vi "experiment control.vi"() -> ()   [LabVIEW 2012] (continued)
  in  "Functions":cluster{"Name":string, "Body":string}[](array[cluster])=[{"Name"="Warmup Ablation Laser", "Body"="Debug: Console >> Start Warmup\nDIO64: Prepare >> Experiment\nFrames >> 50,1\nDIO64: Run\nDebug: Console >> End Warmup"}, {"Name"="Read Wavelengths", "Body"="Wavemeter: Read\nLaser: Read Wavelength >> Lisa"}, {"Name"="scan", "Body"="Begin Scan\n\nScan: Reference >> Disable,All\n\n#Scan: Reference >> Enable,0\n#Scan: Reference >> Enable,1\n#Scan: Reference >> Enable,2\n#Scan: Reference >> Enable,3\n#Scan: Reference >> Enable,4\n#Scan: Reference >> Enable,5\n#Scan: Reference >> Enable,6\n#Scan: Reference >> Enable,7\nScan: Reference >> Enable,8\nScan: Reference >> Enable,9\nScan: Reference >> Enable,10\n\n#Scan: Reset >>0\n#Scan: Reset >>1\n#Scan: Reset >>2\nScan: Reset >>3\n\nFrames  >> 40,40\nScope: Settings >> TDS5034B\nScope: Trigger Settings >> TDS5034B\n\nWhile Loop >> Scan\nTrap DDS: Upload\n\nDAC: Upload2 >> 0,Fast\nFor Loop >> 3\n\nMacro: Clear Wavelengths\nMacro: Read Wavelengths\nQuadDVM: Read\n\nScope: Start >> TDS5034B\nDIO64: Run >> Chop,0\nScope: Read >> TDS5034B\nScope: Stop >> TDS5034B\nScope: Display Traces >> TDS5034B\n\nubinary2 >> Save Scan\n\nEnd Loop\n\n#Scan: Step >>0\n#Scan: Step >>1\n#Scan: Step >>2\nScan: Step >>3\nEnd Loop"}, {"Name"="Scan Experiment Trap Time", "Body"="Frames >> 3,3\nScope: Settings >> TDS5034B\nScope: Trigger Settings >> TDS5034B\n\nBegin Scan\nScan: Reference >> Disable,All\nScan: Reference >> Enable,8\nScan: Reset >> 0\n\nWhile Loop >> Scan\nMacro: Clear Wavelengths\nMacro: Read Wavelengths\n\nScope: Start >> TDS5034B\n\nMV500: Trigger >> True\nDAC: Upload2 >> 1,IMG\nDIO64: Prepare >> 6\nDIO64: Run\nDAC: Upload2 >> 1,Fast\nDIO64: Prepare >> 5\nDIO64: Run\n\nScope: Read >> TDS5034B\nScope: Stop >> TDS5034B\n\nScope: Display Traces >> TDS5034B\nMacro: Read Wavelengths\nuBinary2 >> Save Scan\nScan: Step >> 0\nEnd Loop"}, {"Name"="Scan LIF", "Body"="Frames >> 100, 200\nScope: Settings >> TDS5034B\nScope: Trigger Settings >> TDS5034B\n\nBegin Scan\n\nFor Loop >> 200\nMacro: Clear Wavelengths\nMacro: Read Wavelengths\nScope: Start >> TDS5034B\n#DIO64: Prepare >> Experiment 2-color Photodissoc\nDIO64: Run >> Chop\nScope: Read >> TDS5034B\nScope: Stop >> TDS5034B\nScope: Display Traces >> TDS5034B\nMacro: Read Wavelengths\nuBinary >> Save Scan\nEnd Loop"}, {"Name"="Check ion number", "Body"="Frames >> 30,30\nScope: Settings >> TDS5034B\nScope: Trigger Settings >> TDS5034B\n\nBegin Scan\n\nFor Loop >> 10\nMacro: Clear Wavelengths\nMacro: Read Wavelengths\nCounter: Read\n\nScope: Start >> TDS5034B\nDIO64: Run >> Chop,1\nScope: Read >> TDS5034B\nScope: Stop >> TDS5034B\n\nScope: Display Traces >> TDS5034B\nubinary2 >> Save Scan\nEnd Loop\n"}, {"Name"="Scan Cora", "Body"="Go Today\nMove Down >> scan_cora\n\nFrames >> 15,15\nScope: Settings >> TDS5034B\nScope: Trigger Settings >> TDS5034B\n\nBegin Scan\nLaser: Start Scan >> Cora\nLaser: Step Wavelength >> Cora\nMacro: Read Wavelengths\nWhile Loop >> Cora\nFor Loop >> 3\n\nMacro: Clear Wavelengths\nMacro: Read Wavelengths\nScope: Start >> TDS5034B\nDIO64: Run >> Chop,0\nScope: Read >> TDS5034B\nScope: Stop >> TDS5034B\nScope: Display Traces >> TDS5034B\nMacro: Read Wavelengths\nuBinary: Save\n\nEnd Loop\n\nLaser: Step Wavelength >> Cora\n\nEnd Loop"}, {"Name"="Scan Bertha", "Body"="Frames >> 30,30\nScope: Settings >> TDS5034B\nScope: Trigger Settings >> TDS5034B\n\nBegin Scan\nLaser: Start Scan >> Bertha\nLaser: Step Wavelength >> Bertha\nMacro: Read Wavelengths\nWhile Loop >> Bertha\nFor Loop >> 3\n\nMacro: Clear Wavelengths\nMacro: Read Wavelengths\nScope: Start >> TDS5034B\nDIO64: Run >> Chop,0\nScope: Read >> TDS5034B\nScope: Stop >> TDS5034B\nScope: Display Traces >> TDS5034B\nMacro: Read Wavelengths\nuBinary2 >> Save Scan\n\nEnd Loop\n\nLaser: Step Wavelength >> Bertha\n\nEnd Loop"}, {"Name"="Scan Laser", "Body"="Frames >> 120,120\nScope: Settings >> TDS5034B\nScope: Trigger Settings >> TDS5034B\n\nBegin Scan\nLaser: Start Scan >> TiSapph\nLaser: Step Wavelength >> TiSapph\n\nWhile Loop >> TiSapph\n    For Loop >> 1\n        Scope: Start >> TDS5034B\n        DIO64: Run >> Chop,0\n        Scope: Read >> TDS5034B\n        Scope: Stop >> TDS5034B\n        Scope: Display Traces >> TDS5034B\n        Macro: Clear Wavelengths\n        Macro: Read Wavelengths\nuBinary2 >> Save Scan\n    End Loop\n    Laser: Step Wavelength >> TiSapph\nEnd Loop"}, {"Name"="Scan Toptica", "Body"="Frames >> 30, 30\nScope: Settings >> TDS5034B\nScope: Trigger Settings >> TDS5034B\n\nBegin Scan\n\nScan: Reset All\n\nWhile Loop >> Scan 2\n\nFor Loop >> 5\nMacro: Clear Wavelengths\nMacro: Read Wavelengths\nScope: Start >> TDS5034B\n\nDIO64: Run >> Chop\nScope: Read >> TDS5034B\nScope: Stop >> TDS5034B\nScope: Display Traces >> TDS5034B\nMacro: Read Wavelengths\nuBinary >> Save Scan\nEnd Loop\n\nScan: Step All\nEnd Loop"}, {"Name"="Scan Toptica with DDS reset", "Body"="Frames >> 1,100\nScope: Settings >> TDS5034B\nScope: Trigger Settings >> TDS5034B\n\n\nBegin Scan\n\nScan: Reset All\n\nWhile Loop >> Scan 4\nFor Loop >> 3\n\nMacro: Clear Wavelengths\nMacro: Read Wavelengths\nScope: Start >> TDS5034B\n\nFor Loop >> 50\nTrap DDS: Zero\nTrap DDS: Upload\nDIO64: Prepare >> Experiment 2-color Photodissoc\nDIO64: Run\nTrap DDS: Zero\nTrap DDS: Upload\nDIO64: Prepare >> Experiment 2-color Photodissoc Bkg\nDIO64: Run\nEnd Loop\n\nScope: Read >> TDS5034B\nScope: Stop >> TDS5034B\nScope: Display Traces >> TDS5034B\nMacro: Read Wavelengths\n\nFrames >> 100,100\nuBinary >> Save Scan\nFrames >> 1,100\nEnd Loop\nScan: Step All\nEnd Loop"}, {"Name"="Scan Block", "Body"="For Loop >> 1\n\nBegin Block >> trap_position\nBegin Scan >> Block\nFunction >> Check Position\n\nBegin Block >> scan_switch\nBegin Scan >> Block\nFunction >> Scan Switch\n\nEnd Loop"}, {"Name"="Scan Switch", "Body"="For Loop >> 1\n    Switch: Scan Reset\n    While Loop >> Switch\n    Magnetometer: Measure Background\n    Function >> Scan Ramsey\n    Switch: Scan Step\n    End Loop\nEnd Loop"}, {"Name"="Scan Ramsey", "Body"="Scan: Reference >> Disable,All\nScan: Reference >> Enable,0\nScan: Reference >> Enable,1\nScan: Reference >> Enable,2\nScan: Reference >> Enable,3\n#Scan: Reference >> Enable,4\n\nScan: Reset >> 2\nSwitch: Set >> Doublet\nDAC: Upload2 >> 0,Fast\n\nFrames  >> 4,4\nScope: Settings >> TDS5034B\nScope: Trigger Settings >> TDS5034B\n\nFor Loop >> 1\n    Macro: Clear Wavelengths\n    Macro: Read Wavelengths\n#    QuadDVM: Read\n    Magnetometer: Measure\n\n    Scope: Start >> TDS5034B\n    DIO64: Run >> Chop,1\n    Scope: Read >> TDS5034B\n    Scope: Stop >> TDS5034B\n    Scope: Display Traces >> TDS5034B\n    ubinary2 >> Save Scan\nEnd Loop\n\nWhile Loop >> Scan\n\nFrames  >> 16,16\nScope: Settings >> TDS5034B\nScope: Trigger Settings >> TDS5034B\n\nFor Loop >> 1\n    Macro: Clear Wavelengths\n    Macro: Read Wavelengths\n#    QuadDVM: Read\n    Magnetometer: Measure\n    \n    Scope: Start >> TDS5034B\n    DIO64: Run >> Chop,0\n    Scope: Read >> TDS5034B\n    Scope: Stop >> TDS5034B\n    Scope: Display Traces >> TDS5034B\n    ubinary2 >> Save Scan\nEnd Loop\nScan: Step >> 2\nSwitch: Set >> Doublet\nDAC: Upload2 >> 0,Fast\n   \nEnd Loop"}, {"Name"="Scan Ramsey 2", "Body"="Scan: Reference >> Disable,All\nScan: Reference >> Enable,0\nScan: Reference >> Enable,1\nScan: Reset >> 1\nDAC: Upload2 >> 0,Fast\n\nScan: Reference >> Disable,All\nScan: Reference >> Enable,4\nScan: Reference >> Enable,5\nScan: Reset >> 3\nSwitch: Set >> Doublet\n\nFrames  >> 4,4\nScope: Settings >> TDS5034B\nScope: Trigger Settings >> TDS5034B\n\nFor Loop >> 1\n    Macro: Clear Wavelengths\n    Macro: Read Wavelengths\n    QuadDVM: Read\n    \n    Scope: Start >> TDS5034B\n    DIO64: Run >> Chop,1\n    Scope: Read >> TDS5034B\n    Scope: Stop >> TDS5034B\n    Scope: Display Traces >> TDS5034B\n    ubinary2 >> Save Scan\nEnd Loop\n\nWhile Loop >> Scan\n\nFrames  >> 16,16\nScope: Settings >> TDS5034B\nScope: Trigger Settings >> TDS5034B\n\nFor Loop >> 1\n    Macro: Clear Wavelengths\n    Macro: Read Wavelengths\n    QuadDVM: Read\n    \n    Scope: Start >> TDS5034B\n    DIO64: Run >> Chop,0\n    Scope: Read >> TDS5034B\n    Scope: Stop >> TDS5034B\n    Scope: Display Traces >> TDS5034B\n    ubinary2 >> Save Scan\nEnd Loop\nScan: Step >> 3\nSwitch: Set >> Doublet\n    \nEnd Loop"}, {"Name"="Check Position", "Body"="Scan: Reference >> Disable,All\nScan: Reference >> Enable,0\nScan: Reference >> Enable,1\nScan: Reference >> Enable,2\nScan: Reference >> Enable,3\nScan: Reference >> Enable,4\n\nScan: Reset >> 2\nSwitch: Set >> Doublet\nDAC: Upload2 >> 0,Fast\nUSB DAQ: Digital Write >> 3,1\nUSB DAQ: Digital Write >> 3,0\n\nFrames >> 1,1\nScope: Settings >> TDS5034B\nScope: Trigger Settings >> TDS5034B\n\nScan: Reference >> Disable,All\nScan: Reference >> Enable,8\nScan: Reset >> 0\n\nWhile Loop >> Scan\nMacro: Clear Wavelengths\nMacro: Read Wavelengths\n\nScope: Start >> TDS5034B\n\nMV500: Trigger >> True\nDAC: Upload2 >> 1,IMG\nDIO64: Prepare >> 6\nDIO64: Run\nDAC: Upload2 >> 1,Fast\nDIO64: Prepare >> 5\nDIO64: Run\n\nScope: Read >> TDS5034B\nScope: Stop >> TDS5034B\n\nScope: Display Traces >> TDS5034B\nMacro: Read Wavelengths\nuBinary2 >> Save Scan\nScan: Step >> 0\nEnd Loop\n\nUSB DAQ: Digital Write >> 3,1\nUSB DAQ: Digital Write >> 3,0"}, {"Name"="Scan Pi2", "Body"="Begin Scan\n\nScan: Reference >> Disable,All\nScan: Reference >> Enable,9\nScan: Reset >>1\n\nFrames  >> 20,20\nScope: Settings >> TDS5034B\nScope: Trigger Settings >> TDS5034B\n\nWhile Loop >> Scan\n\nFor Loop >> 4\n    Macro: Clear Wavelengths\n    Macro: Read Wavelengths\n    QuadDVM: Read\n    \n    Scope: Start >> TDS5034B\n    DIO64: Run >> Chop,0\n    Scope: Read >> TDS5034B\n    Scope: Stop >> TDS5034B\n    Scope: Display Traces >> TDS5034B\n    ubinary2 >> Save Scan\nEnd Loop\nScan: Step >> 1\n    \nEnd Loop"}]
  in  "Chop Labels":string[](array[string])=["Antiphase", "Inphase", "Transfer", "Dissociation", "Not Dissociation", "Fast", "IMG"]
  in  "Chops":cluster{"Chops":u16[]}[](array[cluster])=[{"Chops"=[0, 1]}, {"Chops"=[2, 3]}] {"Chops" items=["Antiphase", "Inphase", "Transfer", "Dissociation", "Not Dissociation", "Fast", "IMG"]}
  in  "Channel Labels":T10(array[cluster])=[[{"Channel"="A00:", "Name"="", "plot"=FALSE}, {"Channel"="B00:", "Name"="DDS Ramp 0-1", "plot"=TRUE}, {"Channel"="C00:", "Name"="Unrelax", "plot"=TRUE}, {"Channel"="D00:", "Name"="I/O Update", "plot"=FALSE}], [{"Channel"="A01:", "Name"="Stella AOM shutter", "plot"=FALSE}, {"Channel"="B01:", "Name"="Cora Shutter", "plot"=FALSE}, {"Channel"="C01:", "Name"="Chillax", "plot"=TRUE}, {"Channel"="D01:", "Name"="", "plot"=FALSE}], [{"Channel"="A02:", "Name"="Depletion shutter", "plot"=FALSE}, {"Channel"="B02:", "Name"="DDS Ramp 4-5", "plot"=FALSE}, {"Channel"="C02:", "Name"="", "plot"=FALSE}, {"Channel"="D02:", "Name"="", "plot"=FALSE}], [{"Channel"="A03:", "Name"="Abby Flashlamp", "plot"=FALSE}, {"Channel"="B03:", "Name"="", "plot"=TRUE}, {"Channel"="C03:", "Name"="Trap Gate", "plot"=FALSE}, {"Channel"="D03:", "Name"="", "plot"=FALSE}], [{"Channel"="A04:", "Name"="Abby Q-Switch", "plot"=FALSE}, {"Channel"="B04:", "Name"="End Cap SW0", "plot"=FALSE}, {"Channel"="C04:", "Name"="", "plot"=FALSE}, {"Channel"="D04:", "Name"="", "plot"=FALSE}], [{"Channel"="A05:", "Name"="Img MCP Trigger", "plot"=FALSE}, {"Channel"="B05:", "Name"="266nm Shutter", "plot"=TRUE}, {"Channel"="C05:", "Name"="Change Toptica", "plot"=FALSE}, {"Channel"="D05:", "Name"="", "plot"=FALSE}], [{"Channel"="A06:", "Name"="Trap DDS", "plot"=TRUE}, {"Channel"="B06:", "Name"="B field switch 1", "plot"=FALSE}, {"Channel"="C06:", "Name"="", "plot"=FALSE}, {"Channel"="D06:", "Name"="", "plot"=FALSE}], [{"Channel"="A07:", "Name"="Trigger Scope", "plot"=FALSE}, {"Channel"="B07:", "Name"="B field switch 2", "plot"=FALSE}, {"Channel"="C07:", "Name"="", "plot"=FALSE}, {"Channel"="D07:", "Name"="", "plot"=FALSE}], [{"Channel"="A08:", "Name"="Cora Scan", "plot"=FALSE}, {"Channel"="B08:", "Name"="Trigger Depletion", "plot"=TRUE}, {"Channel"="C08:", "Name"="Far align tool", "plot"=FALSE}, {"Channel"="D08:", "Name"="", "plot"=FALSE}], [{"Channel"="A09:", "Name"="DAC A0", "plot"=FALSE}, {"Channel"="B09:", "Name"="Trigger DAC", "plot"=FALSE}, {"Channel"="C09:", "Name"="", "plot"=FALSE}, {"Channel"="D09:", "Name"="", "plot"=FALSE}], [{"Channel"="A10:", "Name"="DAC A1", "plot"=FALSE}, {"Channel"="B10:", "Name"="DDS Ramp 8-9 ", "plot"=TRUE}, {"Channel"="C10:", "Name"="", "plot"=FALSE}, {"Channel"="D10:", "Name"="", "plot"=FALSE}], [{"Channel"="A11:", "Name"="Toptica Switch", "plot"=TRUE}, {"Channel"="B11:", "Name"="Bertha Scan", "plot"=FALSE}, {"Channel"="C11:", "Name"="", "plot"=FALSE}, {"Channel"="D11:", "Name"="", "plot"=FALSE}], [{"Channel"="A12:", "Name"="End Ramp", "plot"=TRUE}, {"Channel"="B12:", "Name"="DDS Ramp 6-7", "plot"=TRUE}, {"Channel"="C12:", "Name"="", "plot"=FALSE}, {"Channel"="D12:", "Name"="", "plot"=FALSE}], [{"Channel"="A13:", "Name"="Jessica Shutter", "plot"=FALSE}, {"Channel"="B13:", "Name"="End Cap SW1", "plot"=FALSE}, {"Channel"="C13:", "Name"="", "plot"=FALSE}, {"Channel"="D13:", "Name"="", "plot"=FALSE}], [{"Channel"="A14:", "Name"="Gas Pulse Valve", "plot"=FALSE}, {"Channel"="B14:", "Name"="Stella Switch", "plot"=TRUE}, {"Channel"="C14:", "Name"="", "plot"=FALSE}, {"Channel"="D14:", "Name"="", "plot"=FALSE}], [{"Channel"="A15:", "Name"="MCP Framegrabber", "plot"=FALSE}, {"Channel"="B15:", "Name"="Bertha UV Shutter", "plot"=TRUE}, {"Channel"="C15:", "Name"="", "plot"=FALSE}, {"Channel"="D15:", "Name"="", "plot"=FALSE}]]
  in  "USB DAQ":T11={"Digital Out"=[FALSE, FALSE, TRUE, FALSE, FALSE, FALSE, FALSE, FALSE], "Digital In"=[TRUE, TRUE, TRUE, TRUE, TRUE, TRUE, TRUE, TRUE, TRUE, TRUE, TRUE, TRUE, TRUE, TRUE, TRUE, TRUE, TRUE, TRUE, TRUE, TRUE, TRUE, TRUE, TRUE, TRUE, TRUE, TRUE, TRUE, TRUE, TRUE, TRUE, TRUE, TRUE], "Analog Out"=[0, 0], "Analog In"=[0, 0]}
  in  "Chillax":T12={"Chillax"="USB0::0x0957::0x0407::MY44043330::INSTR", "Output"=FALSE, "Chillax Voltage"=0.05, "Unchillax"="USB0::0x0957::0x0407::MY44049806::INSTR"} {"Chillax Voltage" format="%#_6p"}
  in  "Trap Agilent":T13={"USB"="USB0::0x0957::0x0407::MY44031272::INSTR", "Amplitude"=255.0, "Frequency"=50.0, "Phase"=-50.0, "Upload"=FALSE, "Output"=TRUE}
  in  "Depletion Agilent":T14={"USB"="USB0::0x0957::0x2307::MY50003784::INSTR", "Upload"=FALSE, "Output"=TRUE, "Channels"=[{"Frequency"=250000.0, "Phase"=0.0, "Duty Cycle"=10.0, "Trigger"=TRUE}, {"Frequency"=10.0, "Phase"=0.0, "Duty Cycle"=10.0, "Trigger"=FALSE}, {"Frequency"=250.0, "Phase"=121.0, "Duty Cycle"=0.984, "Trigger"=FALSE}, {"Frequency"=250.0, "Phase"=180.0, "Duty Cycle"=1.0, "Trigger"=FALSE}, {"Frequency"=250.0, "Phase"=240.0, "Duty Cycle"=0.992, "Trigger"=FALSE}, {"Frequency"=250.0, "Phase"=300.0, "Duty Cycle"=0.985, "Trigger"=FALSE}, {"Frequency"=250.0, "Phase"=0.0, "Duty Cycle"=0.0, "Trigger"=FALSE}, {"Frequency"=250.0, "Phase"=70.0, "Duty Cycle"=0.0, "Trigger"=FALSE}], "Output Select"=FALSE, "Amplitude"=5.0, "Offset"=2.5} caption="Trap Agilent" {"Channels"."Duty Cycle" min=0.0 max=100.0 step=0.01 format="%#_10g"; "Channels"."Phase" step=0.1 format="%#.2g"; "Channels"."Frequency" format="%#_10p"}
  in  "Coils":T15={"AO Channels"="DAC_COILS/ao0", "DO Lines"="DAC_COILS/port0/line0:1, DAC_COILS/port0/line8", "Keithley USB"="USB0::0x05E6::0x2230::9101029::INSTR", "Current Toggle"=TRUE, "Magnetometer Shim"={"x"=0.023149412102633934, "y"=-0.16449747201584008, "z"=0.07365280387011294, "axgrad"=-0.0001221701881601822}, "Ion Shim"={"x"=0.0, "y"=0.0, "z"=0.0, "axgrad"=0.0}, "Bias"={"x"=0.0, "y"=0.0, "z"=0.0, "axgrad"=0.2563}, "Total"={"x"=0.023149412102633934, "y"=-0.16449747201584008, "z"=0.07365280387011294, "axgrad"=0.2561778298118398}} {"Total"."axgrad" min=-10.0 max=10.0 format="%.5f"; "Total"."z" min=-1.5 max=1.5 step=0.001 format="%.3f"; "Total"."y" min=-1.5 max=1.5 step=0.001 format="%.3f"; "Total"."x" min=-1.5 max=1.5 step=0.001 format="%.3f"; "Bias"."axgrad" min=-10.0 max=10.0 format="%.5f"; "Bias"."z" min=-1.5 max=1.5 step=0.001 format="%.3f"; "Bias"."y" min=-1.5 max=1.5 step=0.001 format="%.3f"; "Bias"."x" min=-1.5 max=1.5 step=0.001 format="%.3f"; "Ion Shim"."axgrad" min=-10.0 max=10.0 format="%.5f"; "Ion Shim"."z" min=-1.5 max=1.5 step=0.001 format="%.3f"; "Ion Shim"."y" min=-1.5 max=1.5 step=0.001 format="%.3f"; "Ion Shim"."x" min=-1.5 max=1.5 step=0.001 format="%.3f"; "Magnetometer Shim"."axgrad" min=-10.0 max=10.0 format="%.5f"; "Magnetometer Shim"."z" min=-1.5 max=1.5 step=0.001 format="%.3f"; "Magnetometer Shim"."y" min=-1.5 max=1.5 step=0.001 format="%.3f"; "Magnetometer Shim"."x" min=-1.5 max=1.5 step=0.001 format="%.3f"}
  in  "Output":T16(tab)=enum."Measurement"
  in  "Jessica":T17={"wavelength"=618.7762925952761, "locked"=TRUE, "lock tolerance"=5e-05, "setpoint"=618.77634, "scan start"=630.8117, "scan end"=632.8217, "progress"=4, "scan step"=7e-05, "scan"=FALSE, "wavelengths"=[]} {"wavelengths" format="%0.6f"; "scan step" format="%#.6g"; "progress" scale=0.0..100.0; "scan end" format="%#.6g"; "scan start" format="%#.6g"; "setpoint" format="%#_9g"; "wavelength" format="%.6g"}
  in  "TiSapph":T18={"wavelength"=814.546398992635, "scan start"=0.755, "scan end"=1.0, "progress"=0, "scan step"=0.02, "scan"=TRUE, "setpoint"=0.855, "wavelengths"=[814.546398992635, 814.546398992635, 814.546398992635, 814.546398992635, 814.546398992635, 814.546398992635, 814.546398992635, 814.546398992635, 814.546398992635, 814.546398992635, 814.546398992635, 814.546398992635, 814.546398992635, 814.546398992635, 814.546398992635, 814.546398992635, 814.546398992635, 814.546398992635, 814.546398992635, 814.546398992635, 814.546398992635, 814.546398992635, 814.546398992635, 814.546398992635, 814.546398992635, 814.546398992635, 814.546398992635, 814.546398992635, 814.546398992635, 814.546398992635, 814.546398992635, 814.546398992635, 814.546398992635, 814.546398992635, 814.546398992635, 814.546398992635, 814.546398992635, 814.546398992635, 814.546398992635, 814.546398992635, 814.546398992635, 814.546398992635, 814.546398992635, 814.546398992635, 814.546398992635, 814.546398992635, 814.546398992635, 814.546398992635, 814.546398992635, 814.546398992635, 814.546398992635, 814.546398992635, 814.546398992635, 814.546398992635, 814.546398992635, 814.546398992635, 814.546398992635, 814.546398992635, 814.546398992635, 814.546398992635, 814.546398992635, 814.546398992635, 814.546398992635, 814.546398992635, 814.546398992635, 814.546398992635, 814.546398992635, 814.546398992635, 814.546398992635, 814.546398992635, 814.546398992635, 814.546398992635, 814.546398992635, 814.546398992635, 814.546398992635, 814.546398992635, 814.546398992635, 814.546398992635, 814.546398992635, 814.546398992635, 814.546398992635, 814.546398992635, 814.546398992635, 814.546398992635, 814.546398992635, 814.546398992635, 814.546398992635, 814.546398992635, 814.546398992635, 814.546398992635, 814.546398992635, 814.546398992635, 814.546398992635, 814.546398992635, 814.546398992635, 814.546398992635, 814.546398992635, 814.546398992635, 814.546398992635, 814.546398992635], "Channel"="DAC_KICK/ao6", "wavelength 2"=12276.771479644609} {"wavelength 2" format="%#.6g"; "wavelengths" format="%0.6f"; "setpoint" format="%#_8g"; "progress" scale=0.0..100.0; "scan end" format="%#_8g"; "scan start" format="%#_8g"; "wavelength" format="%#.6g"}
  in  "Toptica":T19={"wavelength"=986.4230187275185, "locked"=FALSE, "scan start"=899.666791, "scan end"=899.66656, "progress"=52, "scan step"=3e-05, "scan"=TRUE, "AI Channel"="DAC_COILS/ai1"} {"progress" scale=0.0..100.0; "scan end" format="%_10g"; "scan start" format="%.6g"; "wavelength" format="%0.6f"}
  in  "Stella":T20={"wavelength"=899.6693222682825, "locked"=TRUE, "lock tolerance"=5e-06, "setpoint"=0.0, "scan start"=195.0, "scan end"=899.6675, "progress"=0, "scan step"=0.0, "scan"=FALSE, "AI Channel"="DAC_COILS/ai0"} {"progress" scale=0.0..100.0; "setpoint" format="%_10g"; "lock tolerance" format="%.6g"; "wavelength" format="%0.6f"}
  in  "Cora":T21={"wavelength"=817.4773456377446, "locked"=TRUE, "DIO64"="Cora Scan", "scan start"=17987.5, "scan end"=17990.0, "progress"=101, "scan step"=0.04, "scan"=TRUE, "setpoint"=17990.020000000055} {"setpoint" format="%#_8g"; "progress" scale=0.0..100.0; "scan end" format="%#_8g"; "scan start" format="%#_8g"; "wavelength" format="%#.6g"}
  in  "Bertha":T22={"wavelength"=618.7748006391404, "locked"=FALSE, "DIO64"="Bertha Scan", "scan start"=13560.0, "scan end"=13574.0, "progress"=100, "scan step"=0.2, "scan"=FALSE, "setpoint"=13574.000000000051, "wavelengths"=[]} {"wavelengths" format="%0.6f"; "setpoint" format="%#_8g"; "progress" scale=0.0..100.0; "scan end" format="%#_8g"; "scan start" format="%#_8g"; "wavelength" format="%#.6g"}
  in  "Wavemaster":T23={"Serial Port"="COM6", "Wavelength"=13596.86, "Units"="W", "VISA Name"="COM6", "Reading"=FALSE, "Detected"=FALSE} {"Wavelength" format="%_7g"}
  in  "TDS2014 Oscilloscope":T24={"GPIB Address"="GPIB0::2::INSTR", "Detected"=FALSE, "Channels"=[1], "Resolution"=2500, "Frames"=4, "Trigger Position"=0.0, "Trigger Level"=0.01, "Measurements"=[{"Type"="Pk2Pk", "Value"=0.0420000032, "Source"="Ch1"}]} {"Channels" items=["None", "Channel 1", "Channel 2", "Channel 3", "Channel 4", "Math 1", "Math 2", "Math 3", "Math 4", "Reference 1", "Reference 2", "Reference 3", "Reference 4"]}
  in  "TDS5034B Oscilloscope":T24={"GPIB Address"="TCPIP0::192.168.1.102::inst0::INSTR", "Detected"=TRUE, "Channels"=[4], "Resolution"=2500, "Frames"=3, "Trigger Position"=0.0, "Trigger Level"=1.0, "Measurements"=[]} {"Channels" items=["None", "Channel 1", "Channel 2", "Channel 3", "Channel 4", "Math 1", "Math 2", "Math 3", "Math 4", "Reference 1", "Reference 2", "Reference 3", "Reference 4"]}
  out "frames":dbl=1.0
  out "points":i32=2500
  in  "DDS":T25={"address"="USB0::0x0456::0xEE07::NI-VISA-40001::RAW", "channel 1"=350.0, "channel 2"=190.3, "channel 3"=160.0, "channel 4"=185.0, "clock"=23.0, "pll multiplier"=20, "vco gain"=TRUE, "detected"=TRUE, "channel 1 endramp"=330.0, "channel 2 endramp"=200.0, "channel 3 endramp"=0.0, "channel 4 endramp"=185.0, "frequency ramp"=FALSE} {"channel 4 endramp" format="%.9g"; "channel 3 endramp" format="%.9g"; "channel 2 endramp" format="%.9g"; "channel 1 endramp" format="%.9g"; "pll multiplier" max=20; "clock" format="%.9g"; "channel 4" format="%.9g"; "channel 3" format="%.9g"; "channel 2" format="%.9g"; "channel 1" format="%.9g"}
  in  "Trap DDS":T26={"channels"=[{"Frequency"=250.0, "Phase"=0.0, "Amplitude"=0.996}, {"Frequency"=250.0, "Phase"=58.64, "Amplitude"=0.991}, {"Frequency"=250.0, "Phase"=120.56, "Amplitude"=0.984}, {"Frequency"=250.0, "Phase"=179.79, "Amplitude"=1.0}, {"Frequency"=250.0, "Phase"=239.66, "Amplitude"=0.992}, {"Frequency"=250.0, "Phase"=300.48, "Amplitude"=0.985}, {"Frequency"=250.0, "Phase"=0.0, "Amplitude"=0.0}, {"Frequency"=250.0, "Phase"=70.0, "Amplitude"=0.0}], "usb 1"="USB0::0x0456::0xEE07::NI-VISA-70004::RAW", "usb 2"="USB0::0x0456::0xEE07::NI-VISA-60001::RAW", "clock"=10.0, "pll multiplier"=20, "ioupdate"=FALSE, "detected"=TRUE, "ramp"=[{"start"=0.0, "end"=1.0, "ramp time"=200, "edge"=TRUE}, {"start"=1.0, "end"=0.0, "ramp time"=200, "edge"=FALSE}, {"start"=0.0, "end"=1.0, "ramp time"=200, "edge"=TRUE}, {"start"=1.0, "end"=0.0, "ramp time"=15, "edge"=FALSE}, {"start"=0.0, "end"=1.0, "ramp time"=200, "edge"=TRUE}, {"start"=1.0, "end"=0.0, "ramp time"=15, "edge"=FALSE}, {"start"=0.24999999999999997, "end"=1.0, "ramp time"=100, "edge"=FALSE}, {"start"=1.0, "end"=0.24999999999999997, "ramp time"=100, "edge"=TRUE}, {"start"=1.0, "end"=1.0, "ramp time"=200, "edge"=FALSE}, {"start"=1.0, "end"=1.0, "ramp time"=200, "edge"=TRUE}], "232"="COM3", "load ARR"=FALSE, "ramp enable"=FALSE, "ramp time"=100, "Global\nScale Factor"=1.0} {"Global\nScale Factor" min=0.0 max=1.0 step=0.0001 format="%#_10g"; "ramp"."ramp time" max=200 step=1; "ramp"."end" min=0.0 max=1.0 step=0.0001 format="%.3g"; "ramp"."start" min=0.0 max=1.0 step=0.0001 format="%.3g"; "pll multiplier" min=1 max=20; "channels"."Amplitude" min=0.0 max=1.0 step=0.0001 format="%#_10g"; "channels"."Phase" format="%.2f"; "channels"."Frequency" format="%#_10g"}
  in  "HP8341B":T27={"GPIB Port"="GPIB0::19::INSTR", "detected"=FALSE, "rf"=FALSE, "frequency"=-19.5, "stop frequency"=19924.75, "power"=-35.0, "sweep time"=200.0, "Chirp"=TRUE, "Pulse Modulate"=TRUE, "Set frequency"=17924.75} {"sweep time" min=20.0 max=2000.0 step=1.0 format="%#.4f"; "power" min=-100.0 max=-15.0 step=0.01 format="%.2g"; "stop frequency" min=0.0 max=20000.0 step=1e-06 format="%.6g"; "frequency" min=-1000.0 max=1000.0 step=1e-06 format="%.6g"}
  in  "Magnetometer":T28={"Active Boards"=[[{"Status"=TRUE, "Board"="A"}, {"Status"=TRUE, "Board"="B"}, {"Status"=TRUE, "Board"="C"}, {"Status"=TRUE, "Board"="D"}], [{"Status"=TRUE, "Board"="E"}, {"Status"=TRUE, "Board"="F"}, {"Status"=TRUE, "Board"="G"}, {"Status"=TRUE, "Board"="H"}]], "USB ports"=["COM19", "COM20"], "Active Controllers"=[{"Status"=TRUE, "Number"=0.0}, {"Status"=TRUE, "Number"=1.0}], "Measurements"=[]}
  in  "Temperature Monitor":T29={"measurements"=[{"measurement"=6540.75, "location"="Pressure (?)", "label"="Pressure"}, {"measurement"=nan, "location"="Relative Humidity (%)", "label"="Humidity"}, {"measurement"=28.87, "location"="Device Temperature", "label"="Temp"}, {"measurement"=20.5, "location"="inside trap driver", "label"="0x18"}, {"measurement"=24.12, "location"="top gradient coil", "label"="0x19"}, {"measurement"=26.0, "location"="", "label"="0x1A"}, {"measurement"=23.94, "location"="table under chamber", "label"="0x1B"}, {"measurement"=24.0, "location"="diff. pumping flange", "label"="0x1C"}, {"measurement"=23.5, "location"="transfer lasers", "label"="0x1D"}, {"measurement"=nan, "location"="", "label"="0x1E"}, {"measurement"=nan, "location"="", "label"="0x1F"}], "last measurement time"="2015-11-23 01:13:54 PM"}
  in  "Frequency Counter":T30={"GPIB Port"="GPIB0::3::INSTR", "Frequency"=[188789153.79, 0.0, 0.0]} {"Frequency" format="%#_7p"}
  in  "QuadDVM":T31={"Serial Port"="COM5", "Quad DVM"=[[-0.000108], [0.778523], [-0.000129], [0.000241]]} {"Quad DVM" format="%_4f"}
  in  "Scan Variables":T32(array[cluster])=[{"variable"="t", "scan string"="0:0.04:2", "randomize"=FALSE, "enable"=FALSE}, {"variable"="t", "scan string"=".2:0.025:0.8", "randomize"=FALSE, "enable"=FALSE}, {"variable"="t1", "scan string"="0.1:8:56.1 100:16:156 200:8:256", "randomize"=FALSE, "enable"=TRUE}, {"variable"="t1", "scan string"="0.5 1 2 4 6", "randomize"=FALSE, "enable"=FALSE}, {"variable"="x", "scan string"="0", "randomize"=FALSE, "enable"=FALSE}, {"variable"="x", "scan string"="0", "randomize"=FALSE, "enable"=FALSE}]
  in  "Scan References":T33(array[cluster])=[{"scan"=FALSE, "Reference"="End Trap", "equation"="ceil((t+10)/100)*100 + 200.12", "index"=0, "progress"=0, "next"=300.12}, {"scan"=FALSE, "Reference"="DAC Dissociation", "equation"="ceil((t+10)/100)*100 + 99", "index"=0, "progress"=0, "next"=199.0}, {"scan"=FALSE, "Reference"="Doublet Lower T", "equation"="t1", "index"=0, "progress"=0, "next"=8.1}, {"scan"=FALSE, "Reference"="Doublet Upper T", "equation"="t1", "index"=0, "progress"=0, "next"=8.1}, {"scan"=FALSE, "Reference"="DAC Return", "equation"="t1 + 6 + 114 + 1.28*2", "index"=0, "progress"=0, "next"=130.66}, {"scan"=FALSE, "Reference"="End Pi/2 Pulse", "equation"="t1", "index"=0, "progress"=0, "next"=16.0}, {"scan"=FALSE, "Reference"="Brot", "equation"="t", "index"=26, "progress"=100, "next"=0.1}, {"scan"=FALSE, "Reference"="End DDS Ramp 1", "equation"="t2 - 280", "index"=0, "progress"=0, "next"=220.0}, {"scan"=TRUE, "Reference"="End Trap", "equation"="t+118", "index"=0, "progress"=0, "next"=126.1}, {"scan"=FALSE, "Reference"="End Trigger Depletion 2", "equation"="t", "index"=5, "progress"=100, "next"=6.0}, {"scan"=FALSE, "Reference"="End Trigger Depletion 2-dephase", "equation"="t", "index"=5, "progress"=100, "next"=6.0}, {"scan"=FALSE, "Reference"="End Trap", "equation"="600.14 + t", "index"=0, "progress"=0, "next"=606.48}] {"progress" scale=0.0..100.0}
  in  "Clear IMG MCP":bool=TRUE
  in  "img_mcp:averages":u32=3 caption="Averages"
  out "img mcp":dbl[][](graph) caption="IMG MCP"
  in  "Column":u32=1
  out "DIO64 Graph":cluster{dbl[], dbl[]}[](graph)=[{[0.0, 0.1720000000000006, 6.09301, 6.103010000000001, 18.174400000000002, 18.1844, 19.172, 19.182000000000002, 19.3181, 19.328100000000003, 19.383100000000002, 19.4432, 19.453200000000002, 20.131, 20.171, 20.172, 24.073, 24.078, 24.083000000000002, 24.088, 24.09301, 24.098, 24.10301, 34.078, 100.172], [0.0, 0.0, 0.0, 0.0, 0.0, 0.0, 0.0, 0.0, 0.0, 0.0, 0.0, 0.0, 0.0, 0.0, 0.0, 1.0, 0.0, 0.0, 0.0, 0.0, 0.0, 0.0, 0.0, 0.0, 0.0]}, {[0.0, 0.1720000000000006, 6.09301, 6.103010000000001, 18.174400000000002, 18.1844, 19.172, 19.182000000000002, 19.3181, 19.328100000000003, 19.383100000000002, 19.4432, 19.453200000000002, 20.131, 20.171, 20.172, 24.073, 24.078, 24.083000000000002, 24.088, 24.09301, 24.098, 24.10301, 34.078, 100.172], [-1.2, -1.2, -1.2, -1.2, -1.2, -1.2, -1.2, -1.2, -1.2, -1.2, -1.2, -1.2, -1.2, -1.2, -1.2, -1.2, -1.2, -1.2, -1.2, -1.2, -1.2, -1.2, -1.2, -1.2, -1.2]}, {[0.0, 0.1720000000000006, 6.09301, 6.103010000000001, 18.174400000000002, 18.1844, 19.172, 19.182000000000002, 19.3181, 19.328100000000003, 19.383100000000002, 19.4432, 19.453200000000002, 20.131, 20.171, 20.172, 24.073, 24.078, 24.083000000000002, 24.088, 24.09301, 24.098, 24.10301, 34.078, 100.172], [-2.4, -2.4, -2.4, -2.4, -2.4, -2.4, -2.4, -2.4, -2.4, -2.4, -2.4, -2.4, -2.4, -2.4, -2.4, -2.4, -2.4, -2.4, -2.4, -2.4, -2.4, -2.4, -2.4, -2.4, -2.4]}, {[0.0, 0.1720000000000006, 6.09301, 6.103010000000001, 18.174400000000002, 18.1844, 19.172, 19.182000000000002, 19.3181, 19.328100000000003, 19.383100000000002, 19.4432, 19.453200000000002, 20.131, 20.171, 20.172, 24.073, 24.078, 24.083000000000002, 24.088, 24.09301, 24.098, 24.10301, 34.078, 100.172], [-3.5999999999999996, -3.5999999999999996, -3.5999999999999996, -3.5999999999999996, -3.5999999999999996, -3.5999999999999996, -3.5999999999999996, -3.5999999999999996, -3.5999999999999996, -3.5999999999999996, -3.5999999999999996, -3.5999999999999996, -3.5999999999999996, -3.5999999999999996, -3.5999999999999996, -3.5999999999999996, -3.5999999999999996, -3.5999999999999996, -3.5999999999999996, -3.5999999999999996, -3.5999999999999996, -3.5999999999999996, -3.5999999999999996, -3.5999999999999996, -3.5999999999999996]}, {[0.0, 0.1720000000000006, 6.09301, 6.103010000000001, 18.174400000000002, 18.1844, 19.172, 19.182000000000002, 19.3181, 19.328100000000003, 19.383100000000002, 19.4432, 19.453200000000002, 20.131, 20.171, 20.172, 24.073, 24.078, 24.083000000000002, 24.088, 24.09301, 24.098, 24.10301, 34.078, 100.172], [-4.8, -4.8, -4.8, -4.8, -4.8, -4.8, -4.8, -4.8, -4.8, -4.8, -4.8, -4.8, -4.8, -4.8, -4.8, -4.8, -4.8, -4.8, -4.8, -4.8, -4.8, -4.8, -4.8, -4.8, -4.8]}, {[0.0, 0.1720000000000006, 6.09301, 6.103010000000001, 18.174400000000002, 18.1844, 19.172, 19.182000000000002, 19.3181, 19.328100000000003, 19.383100000000002, 19.4432, 19.453200000000002, 20.131, 20.171, 20.172, 24.073, 24.078, 24.083000000000002, 24.088, 24.09301, 24.098, 24.10301, 34.078, 100.172], [-6.0, -6.0, -6.0, -6.0, -6.0, -6.0, -6.0, -6.0, -6.0, -6.0, -6.0, -6.0, -6.0, -6.0, -6.0, -6.0, -6.0, -6.0, -6.0, -6.0, -6.0, -6.0, -6.0, -6.0, -6.0]}, {[0.0, 0.1720000000000006, 6.09301, 6.103010000000001, 18.174400000000002, 18.1844, 19.172, 19.182000000000002, 19.3181, 19.328100000000003, 19.383100000000002, 19.4432, 19.453200000000002, 20.131, 20.171, 20.172, 24.073, 24.078, 24.083000000000002, 24.088, 24.09301, 24.098, 24.10301, 34.078, 100.172], [-7.2, -7.2, -7.2, -7.2, -7.2, -7.2, -7.2, -7.2, -7.2, -7.2, -7.2, -7.2, -7.2, -7.2, -7.2, -7.2, -7.2, -7.2, -7.2, -7.2, -7.2, -7.2, -7.2, -7.2, -7.2]}, {[0.0, 0.1720000000000006, 6.09301, 6.103010000000001, 18.174400000000002, 18.1844, 19.172, 19.182000000000002, 19.3181, 19.328100000000003, 19.383100000000002, 19.4432, 19.453200000000002, 20.131, 20.171, 20.172, 24.073, 24.078, 24.083000000000002, 24.088, 24.09301, 24.098, 24.10301, 34.078, 100.172], [-8.4, -8.4, -8.4, -8.4, -8.4, -8.4, -8.4, -8.4, -8.4, -8.4, -8.4, -8.4, -8.4, -8.4, -8.4, -8.4, -8.4, -8.4, -8.4, -8.4, -8.4, -8.4, -8.4, -8.4, -8.4]}, {[0.0, 0.1720000000000006, 6.09301, 6.103010000000001, 18.174400000000002, 18.1844, 19.172, 19.182000000000002, 19.3181, 19.328100000000003, 19.383100000000002, 19.4432, 19.453200000000002, 20.131, 20.171, 20.172, 24.073, 24.078, 24.083000000000002, 24.088, 24.09301, 24.098, 24.10301, 34.078, 100.172], [-9.6, -9.6, -9.6, -9.6, -9.6, -9.6, -9.6, -9.6, -9.6, -9.6, -9.6, -9.6, -9.6, -9.6, -9.6, -9.6, -9.6, -9.6, -9.6, -9.6, -9.6, -9.6, -9.6, -9.6, -9.6]}, {[0.0, 0.1720000000000006, 6.09301, 6.103010000000001, 18.174400000000002, 18.1844, 19.172, 19.182000000000002, 19.3181, 19.328100000000003, 19.383100000000002, 19.4432, 19.453200000000002, 20.131, 20.171, 20.172, 24.073, 24.078, 24.083000000000002, 24.088, 24.09301, 24.098, 24.10301, 34.078, 100.172], [-10.799999999999999, -10.799999999999999, -10.799999999999999, -10.799999999999999, -10.799999999999999, -10.799999999999999, -10.799999999999999, -10.799999999999999, -10.799999999999999, -10.799999999999999, -10.799999999999999, -10.799999999999999, -10.799999999999999, -10.799999999999999, -10.799999999999999, -10.799999999999999, -10.799999999999999, -10.799999999999999, -10.799999999999999, -10.799999999999999, -10.799999999999999, -10.799999999999999, -10.799999999999999, -10.799999999999999, -10.799999999999999]}, {[0.0, 0.1720000000000006, 6.09301, 6.103010000000001, 18.174400000000002, 18.1844, 19.172, 19.182000000000002, 19.3181, 19.328100000000003, 19.383100000000002, 19.4432, 19.453200000000002, 20.131, 20.171, 20.172, 24.073, 24.078, 24.083000000000002, 24.088, 24.09301, 24.098, 24.10301, 34.078, 100.172], [-11.999999999999998, -10.999999999999998, -10.999999999999998, -10.999999999999998, -10.999999999999998, -10.999999999999998, -10.999999999999998, -10.999999999999998, -10.999999999999998, -10.999999999999998, -10.999999999999998, -10.999999999999998, -10.999999999999998, -10.999999999999998, -10.999999999999998, -10.999999999999998, -10.999999999999998, -10.999999999999998, -10.999999999999998, -10.999999999999998, -10.999999999999998, -10.999999999999998, -10.999999999999998, -10.999999999999998, -11.999999999999998]}, {[0.0, 0.1720000000000006, 6.09301, 6.103010000000001, 18.174400000000002, 18.1844, 19.172, 19.182000000000002, 19.3181, 19.328100000000003, 19.383100000000002, 19.4432, 19.453200000000002, 20.131, 20.171, 20.172, 24.073, 24.078, 24.083000000000002, 24.088, 24.09301, 24.098, 24.10301, 34.078, 100.172], [-13.199999999999998, -13.199999999999998, -13.199999999999998, -13.199999999999998, -13.199999999999998, -13.199999999999998, -13.199999999999998, -13.199999999999998, -13.199999999999998, -13.199999999999998, -13.199999999999998, -13.199999999999998, -13.199999999999998, -13.199999999999998, -13.199999999999998, -13.199999999999998, -13.199999999999998, -13.199999999999998, -13.199999999999998, -13.199999999999998, -13.199999999999998, -13.199999999999998, -13.199999999999998, -13.199999999999998, -13.199999999999998]}, {[0.0, 0.1720000000000006, 6.09301, 6.103010000000001, 18.174400000000002, 18.1844, 19.172, 19.182000000000002, 19.3181, 19.328100000000003, 19.383100000000002, 19.4432, 19.453200000000002, 20.131, 20.171, 20.172, 24.073, 24.078, 24.083000000000002, 24.088, 24.09301, 24.098, 24.10301, 34.078, 100.172], [-14.399999999999997, -14.399999999999997, -14.399999999999997, -14.399999999999997, -14.399999999999997, -14.399999999999997, -14.399999999999997, -14.399999999999997, -14.399999999999997, -14.399999999999997, -14.399999999999997, -14.399999999999997, -14.399999999999997, -14.399999999999997, -14.399999999999997, -14.399999999999997, -14.399999999999997, -14.399999999999997, -14.399999999999997, -14.399999999999997, -14.399999999999997, -14.399999999999997, -14.399999999999997, -14.399999999999997, -14.399999999999997]}]
  in  "Count Ions":T34={"Hf  time threshold"=4.85e-06, "Ion Calibration"=1.05e-09, "Hf integrated"=4.094171428571428, "HfF"=313.92487619047574, "Hf integrated history"=[4.094171428571428, 4.094171428571428, -2.873295238095233, -2.873295238095233, -0.35230476190476234, -0.35230476190476234, -1.2318476190476184, -1.2318476190476184, 1.46712380952381, 1.46712380952381, -2.4691809523809507, -2.4691809523809507, 0.5156571428571459, 0.5156571428571459, 2.3533714285714313, 2.3533714285714313, -0.13470476190476538, -0.13470476190476538, -1.6335238095238096, -1.6335238095238096], "HfF history"=[313.92487619047574, 313.92487619047574, 442.41615238095216, 442.41615238095216, 243.70468571428606, 243.70468571428606, 479.9366095238095, 479.9366095238095, 531.9423999999988, 531.9423999999988, 473.0215619047611, 473.0215619047611, 366.6462476190471, 366.6462476190471, 222.8656761904756, 222.8656761904756, 336.515657142858, 336.515657142858, 356.0716190476186, 356.0716190476186], "<Hf integrated>"=-0.026453333333332392, "<HfF>"=376.70454857142823, "XY Graph"=[], "History"=20, "Clear History"=FALSE}
  out "stdout":string="\r\n****************************\r\n**  Starting Experiment Control  **\r\n****************************\r\n2015-11-23 01:10 PM: VISA Write in Wmeter Initialize.vi->experiment control.vi\r\nCan't Find Wavemeter\r\nInitializing Scope TDS5034B\r\n2015-11-23 01:10 PM: VISA Write in experiment control.vi\r\nInitializing Scope TDS2014\r\n2015-11-23 01:10 PM: Agilent 33XXX Series.lvlib:Initialize.vi<ERR>\nThe ID Query failed.  This may mean that you selected the wrong instrument or your instrument did not respond.  You may also be using a model that is not officially supported by this driver.  If you are sure that you have selected the correct instrument and it is responding, try disabling the ID Query.\n\n\n<b>Complete call chain:</b>\r\n     Agilent 33XXX Series.lvlib:Initialize.vi\r\n     experiment control.vi\r\nInitializing Wavemeter\r\nInitializing DIO64\r\n****************************\r\n**  Exiting Experiment Control  **\r\n****************************\r\nClosing DIO64"
  out "debug timing":cluster{"command":string, "time":dbl}[](array[cluster])=[{"command"="Exit", "time"=0.0}, {"command"="Data: Initialize", "time"=0.0}, {"command"="Data: Cleanup", "time"=0.0}, {"command"="UI: Initialize", "time"=0.0}, {"command"="UI: Cursor Set", "time"=0.0}, {"command"="UI: Front Panel State", "time"=0.0}, {"command"="UI: DIO64 Update Control", "time"=21.0}, {"command"="UI: Update Scan References", "time"=2.0}, {"command"="UI: Update State Hierarchy", "time"=0.0}, {"command"="UI: DIO64 Change Labels", "time"=16.0}, {"command"="UI: Chop Labels", "time"=0.0}, {"command"="UI: DAC Update Listing", "time"=8.0}, {"command"="UI: DAC Update Graph2", "time"=0.0}, {"command"="UI: Get Case Strings", "time"=0.0}, {"command"="UI: Get Case Documentation", "time"=0.0}, {"command"="Macro: Initialize", "time"=0.0}, {"command"="Macro: Read Wavelengths", "time"=0.0}, {"command"="Macro: Exit", "time"=7.0}, {"command"="Function", "time"=0.0}, {"command"="Clear", "time"=0.0}, {"command"="Abort", "time"=0.0}, {"command"="Test", "time"=0.0}, {"command"="Pause", "time"=0.0}, {"command"="Unpause", "time"=0.0}, {"command"="Wait", "time"=0.0}, {"command"="Sync", "time"=0.0}, {"command"="Tick", "time"=0.0}, {"command"="Tock", "time"=0.0}, {"command"="For Loop", "time"=0.0}, {"command"="While Loop", "time"=0.0}, {"command"="Count Ions", "time"=0.0}, {"command"="uBinary: Save", "time"=0.0}, {"command"="uBinary: Load", "time"=0.0}, {"command"="uBinary2", "time"=0.0}, {"command"="Begin Block", "time"=0.0}, {"command"="Next Block", "time"=0.0}, {"command"="Begin Scan", "time"=0.0}, {"command"="Frames", "time"=0.0}, {"command"="Scope: Frames", "time"=0.0}, {"command"="DIO64: Frames", "time"=0.0}, {"command"="MV500: Trigger", "time"=0.0}, {"command"="IMG MCP: Clear", "time"=0.0}, {"command"="MV500: Read", "time"=0.0}, {"command"="Move Down", "time"=0.0}, {"command"="Move Up", "time"=0.0}, {"command"="Go Today", "time"=0.0}, {"command"="Check Lasers", "time"=0.0}, {"command"="Depletion Flip", "time"=0.0}, {"command"="Bertha Flip", "time"=0.0}, {"command"="Switch: Scan Reset", "time"=0.0}, {"command"="Switch: Scan Step", "time"=0.0}, {"command"="Switch: Set Machine State", "time"=0.0}, {"command"="Switch: Set", "time"=0.0}, {"command"="Switch: Change State", "time"=0.0}, {"command"="Switch: Update Hierarchy", "time"=0.0}, {"command"="Scan: Step", "time"=0.0}, {"command"="Scan: Reset", "time"=0.0}, {"command"="Scan: Reference", "time"=0.0}, {"command"="Laser: Step Wavelength", "time"=0.0}, {"command"="Laser: Start Scan", "time"=0.0}, {"command"="Laser: Read Wavelength", "time"=0.0}, {"command"="Laser: Initialize DAC", "time"=1.0}, {"command"="Laser: Close DAC", "time"=1.0}, {"command"="Debug: Popup", "time"=0.0}, {"command"="Debug: Console", "time"=1.0}, {"command"="Wavemeter: Initialise", "time"=1657.0}, {"command"="Wavemeter: Start", "time"=0.0}, {"command"="Wavemeter: Set Units", "time"=0.0}, {"command"="Wavemeter: Read", "time"=0.0}, {"command"="Wavemeter: Stop", "time"=0.0}, {"command"="Wavemeter: Close", "time"=0.0}, {"command"="DIO64: Initialise", "time"=2033.0}, {"command"="DIO64: Prepare", "time"=0.0}, {"command"="DIO64: Update Graph", "time"=0.0}, {"command"="DIO64: Run", "time"=0.0}, {"command"="DIO64: Override", "time"=0.0}, {"command"="DIO64: Trigger", "time"=0.0}, {"command"="DIO64: Close", "time"=1.0}, {"command"="Scope: Initialise", "time"=1.0}, {"command"="Scope: Start", "time"=0.0}, {"command"="Scope: Read", "time"=0.0}, {"command"="Scope: Settings", "time"=0.0}, {"command"="Scope: Trigger Settings", "time"=0.0}, {"command"="Scope: Measurement Settings", "time"=0.0}, {"command"="Scope: Measurement", "time"=0.0}, {"command"="Scope: Display Traces", "time"=0.0}, {"command"="Scope: Stop", "time"=0.0}, {"command"="Scope: Close", "time"=0.0}, {"command"="Trap DDS: Set Clock", "time"=1.0}, {"command"="Trap DDS: IOUpdate", "time"=0.0}, {"command"="Trap DDS: Upload", "time"=6.0}, {"command"="Trap DDS: Upload Ramp", "time"=0.0}, {"command"="Trap DDS: Connect Serial", "time"=4.0}, {"command"="Trap DDS: Disconnect Serial", "time"=0.0}, {"command"="Trap DDS: Zero", "time"=0.0}, {"command"="Trap DDS: Reset", "time"=0.0}, {"command"="DDS: Set Clock", "time"=5.0}, {"command"="DDS: Set Frequency Ramp", "time"=0.0}, {"command"="DDS: Set Frequency", "time"=4.0}, {"command"="DDS: Goto Frequency", "time"=10.0}, {"command"="Coils: Initialize", "time"=4432.0}, {"command"="Coils: Close", "time"=20.0}, {"command"="Coils: Set", "time"=34.0}, {"command"="DAC: Upload2", "time"=0.0}, {"command"="DAC: View", "time"=0.0}, {"command"="DAC: Clear", "time"=0.0}, {"command"="Depletion Agilent: Initialize", "time"=43.0}, {"command"="Depletion Agilent: Set", "time"=4.0}, {"command"="Depletion Agilent: Output", "time"=0.0}, {"command"="Depletion Agilent: Close", "time"=1.0}, {"command"="Chillax: Initialize", "time"=335.0}, {"command"="Chillax: Close", "time"=0.0}, {"command"="Chillax: Set Voltage", "time"=0.0}, {"command"="Chillax: Output", "time"=0.0}, {"command"="Trap Agilent: Initialize", "time"=131.0}, {"command"="Trap Agilent: Set", "time"=184.0}, {"command"="Trap Agilent: Output", "time"=0.0}, {"command"="Trap Agilent: Close", "time"=3.0}, {"command"="USB DAQ: Initialize", "time"=19.0}, {"command"="USB DAQ: Digital Write", "time"=4.0}, {"command"="USB DAQ: Digital Read", "time"=0.0}, {"command"="USB DAQ: Analog Write", "time"=0.0}, {"command"="USB DAQ: Analog Read", "time"=0.0}, {"command"="QuadDVM: Initialize", "time"=16.0}, {"command"="QuadDVM: Read", "time"=0.0}, {"command"="QuadDVM: Close", "time"=425.0}, {"command"=" ------- Temperature Monitor -------", "time"=0.0}, {"command"="Temperature: Read", "time"=0.0}, {"command"=" ------- Magnetometer -------", "time"=0.0}, {"command"="Magnetometer: Initialize", "time"=6973.0}, {"command"="Magnetometer: Read", "time"=0.0}, {"command"="Magnetometer: Close", "time"=0.0}, {"command"="Counter: Initialize", "time"=0.0}, {"command"="Counter: Read", "time"=0.0}, {"command"="Counter: Close", "time"=0.0}, {"command"="Microwave: Setup", "time"=0.0}, {"command"="Microwave: RF", "time"=0.0}, {"command"="Microwave: Pulse", "time"=0.0}, {"command"="Microwave: Set Frequency", "time"=0.0}, {"command"="Microwave: Set Power", "time"=0.0}, {"command"="Microwave: Set Sweep Time", "time"=0.0}, {"command"="Microwave: Set Sweep", "time"=0.0}] caption="Debug Timing"
  out "queue":string[](array[string])
  in  "update_debug":bool
  in  "DIO64 Override":T35={"DIO64 Line 1"=[FALSE, FALSE, FALSE, FALSE, FALSE, FALSE, FALSE, FALSE, FALSE, FALSE, FALSE, FALSE, FALSE, FALSE, FALSE, FALSE], "DIO64 Line 2"=[FALSE, FALSE, FALSE, FALSE, FALSE, FALSE, TRUE, FALSE, FALSE, FALSE, FALSE, FALSE, FALSE, FALSE, FALSE, FALSE], "DIO64 Line 3"=[FALSE, FALSE, FALSE, FALSE, FALSE, FALSE, FALSE, FALSE, FALSE, FALSE, FALSE, FALSE, FALSE, FALSE, FALSE, FALSE], "DIO64 Line 4"=[FALSE, FALSE, FALSE, FALSE, FALSE, FALSE, FALSE, FALSE, FALSE, FALSE, FALSE, FALSE, FALSE, FALSE, FALSE, FALSE]}
